vi "Configure Trigger E Source.vi"(8 "error in (no error)":errorcluster, 9 "Source (\"No Connection\")":string="No Connection", 10 "Trigger (1)":i32=1, 11 "VISA resource name":refnum<visa-resource-name>) -> (0 "error out":errorcluster, 3 "VISA resource name out":refnum<visa-resource-name>)   [LabVIEW 2020, in "Rohde&Schwarz CMXP Base.lvlib"]
doc: "Selects the output trigger signals to be routed to the trigger connectors. A list of all supported values can be retrieved using RSCMXPBASE_ATTR_TRIGGER_E_SOURCE_CATALOG.\n\nAttributes:\nRSCMXPBASE_ATTR_SELECT_TRIGGER\nRSCMXPBASE_ATTR_TRIGGER_E_SOURCE\n\nRemote-control command:\nTRIGger:BASE:EXTE<n>:SOURce"
uses:
  <instrlib>/Rohde&Schwarz CMXP Base/Rohde&Schwarz CMXP Base.lvlib
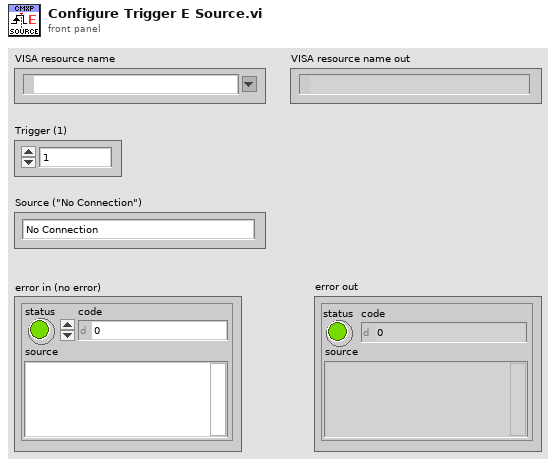
[diagram p1: front panel]
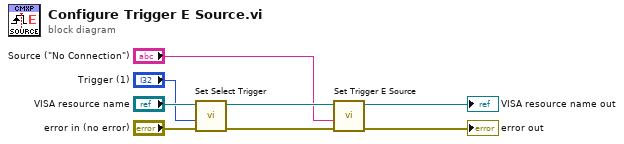
[diagram p0: block diagram]
diagram:
  n1 = call "Set Select Trigger"("error in (no error)"="error in (no error)", "Select Trigger (0)"="Trigger (1)", "instrument handle"="VISA resource name") -> ("error out"=w3:errorcluster, "instrument handle out"=w4:refnum<visa-resource-name>)  [unwired: 7 in]
  n2 = call "Set Trigger E Source"("error in (no error)"=w3, "Trigger E Source ()"="Source (\"No Connection\")", "instrument handle"=w4) -> ("error out"=→"error out":errorcluster, "instrument handle out"=→"VISA resource name out":refnum<visa-resource-name>)  [unwired: 7 in]
